vi "Create (Single).vi"(7 "Correction Level (Default: Level L)":T1, 8 "error in (no error)":errorcluster) -> (0 "error out":errorcluster, 3 "QR Code Encoder":refnum<class "QR Code Encoder.lvclass">)   [LabVIEW 2020, in "feature_detection.lvlib" / "QR Code Encoder.lvclass"]
doc: "Create a QR Code Generator."
uses:
  QR Code Encoder.lvclass
  Correction Levels.ctl
  QR Code Encoder.lvclass/QR Code Encoder.ctl
  <vilib>/Utility/error.llb/Error Cluster From Error Code.vi
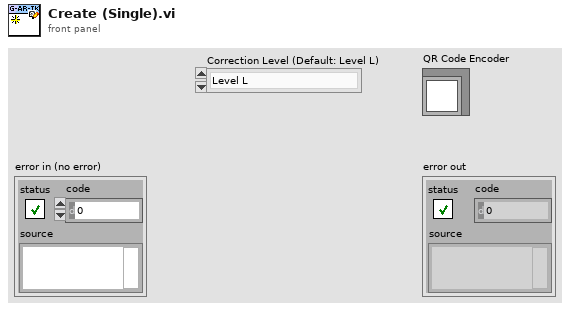
[diagram p1: front panel]
types:
  T1 = typedef "feature_detection.lvlib/QR Code Encoder.lvclass/Correction Levels.ctl" = enum16{"Level L", "Level M", "Level Q", "Level H"}
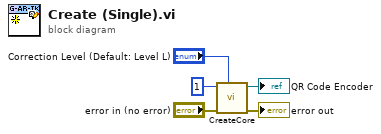
[diagram p0: block diagram]
diagram:
  n1 = call "CreateCore.vi"("Correction Levels"="Correction Level (Default: Level L)", "error in (no error)"="error in (no error)", "n_qr_codes"=u8 1) -> ("error out"=→"error out":errorcluster, "QR Code Encoder"=→"QR Code Encoder":refnum<class "QR Code Encoder.lvclass">)  [unwired: 7 in]
